vi "asfasaf.vi"() -> ()   [LabVIEW 2019]
uses:
  <vilib>/Utility/file.llb/Write Delimited Spreadsheet (string).vi
panel:
  in  "error in":errorcluster
  out "appended path":path
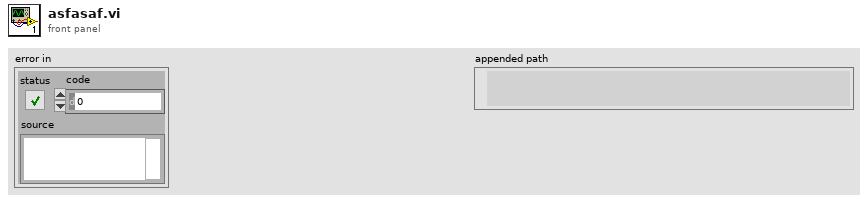
[diagram p1: front panel]
types:
  T1 = enum16{"open", "replace", "create", "open or create", "replace or create", "replace or create with confirmation"}
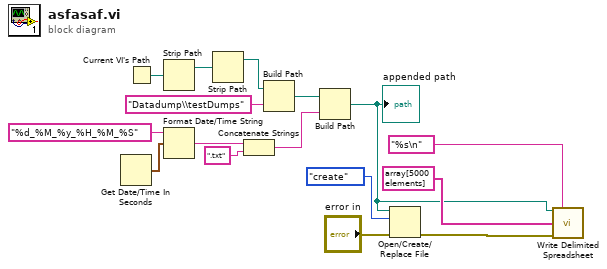
[diagram p0: block diagram]
diagram:
  n1 = Get Date/Time In Seconds() -> (seconds since 1Jan1904=w14:timestamp)
  n2 = Current VI's Path() -> (path=w16:path)
  n3 = Strip Path(path=w16) -> (stripped path=w3:path)  [unwired: 1 out]
  n4 = Format Date/Time String(time format string (%c)="%d_%M_%y_%H_%M_%S", seconds (now)=w14) -> (date/time string=w11:string)  [unwired: 1 in]
  n5 = Strip Path(path=w3) -> (stripped path=w2:path)  [unwired: 1 out]
  n6 = Concatenate Strings(w11, ".txt") -> (w9:string)
  n7 = Build Path(base path=w2, name or relative path="Datadump\\testDumps") -> (appended path=w12:path)
  n8 = Build Path(base path=w12, name or relative path=w9) -> (appended path=w1:path)
  "appended path" <- w1
  n9 = Open/Create/Replace File(file path (use dialog)=w1, error in="error in", operation (0:open)=T1."create") -> (error out=w6:errorcluster)  [unwired: 3 in, 2 out]
  n10 = call-poly <vilib>:"Write Delimited Spreadsheet.vi"("file path (dialog if empty)"=w1, "format (%s)"="%s\n", "1D data"=string[] array[5000 elements] ("Array"), "error in (no error)"=w6) -> ()  [unwired: 10 in, 2 out]
